vi "Attributes Setup.vi"(11 "IMAQdx Cam in":refnum<class "IMAQdx Cam.lvclass">) -> ()   [LabVIEW 2009, in "IMAQdx Cam.lvclass"]
doc: "The Grab and Attributes Setup example VI allows the user to view the current attributes and settings, update attribute settings, acquire images continuously, and display the images in an image control."
uses:
  IMAQdx Cam.lvclass
  IMAQdx Cam.lvclass/IMAQdx Cam.ctl
panel:
  in  "Filter":string
  in  "error in":errorcluster
  out "Tooltip":string
  out "Units":string
  out "Tab Control Ref":T1
  in  "Tab Control":T2(tab)
  in  "U32 Value Control":u32(slide) scale=4.0..4044.0
  in  "DBL Value Control":dbl(slide) min=17.00000029813964 max=5000000.0 step=1.0 scale=17.00000029813964..5000000.0
  in  "String Value Control":string
  in  "Enum Value Control":u32(ring) items=["Use hardware value", "10-bit", "12-bit", "14-bit", "16-bit"]
  in  "Boolean Value Control":bool=TRUE
  in  "Command Value Control":bool
  in  "Attribute Table":string(tree)
  in  "stop":bool
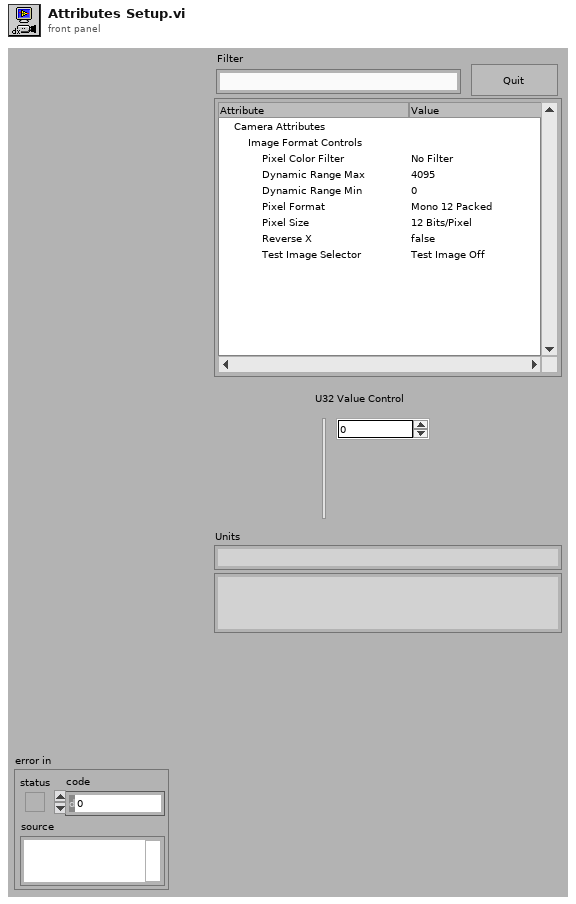
[diagram p1: front panel]
types:
  T1 = cluster{"Tab Control":refnum<vi>, "U32 Value Control":refnum<vi>, "DBL Value Control":refnum<vi>, "String Value Control":refnum<vi>, "Enum Value Control":refnum<vi>, "Boolean Value Control":refnum<vi>, "Command Value Control":refnum<vi>}
  T2 = enum32{"U32", "DBL", "String", "Enum", "Bool", "Command"}
  T3 = typedef "IMAQdx.ctl" = refnum<k21>
  T4 = typedef "eventvkey.ctl" = enum16{"ASCII", "Enter", "Return", "Shift", "Ctrl", "Alt", "Cmd", "Opt", "Caps", "NumLock", "Clear", "Break", "Up", "Down", "Left", "Right", "Insert", "Delete", "Home", "End", "PageUp", "PageDown", "Escape", "Help", "Pause", "ScrollLock", "F1", "F2", "F3", "F4", "F5", "F6", "F7", "F8", "F9", "F10", "F11", "F12", "F13", "F14", "F15", "F16", "F17", "F18", "F19", "F20", "F21", "F22", "F23", "F24", "Play", "VolumeUp", "VolumeDown", "Mute", "Two Byte Char"}
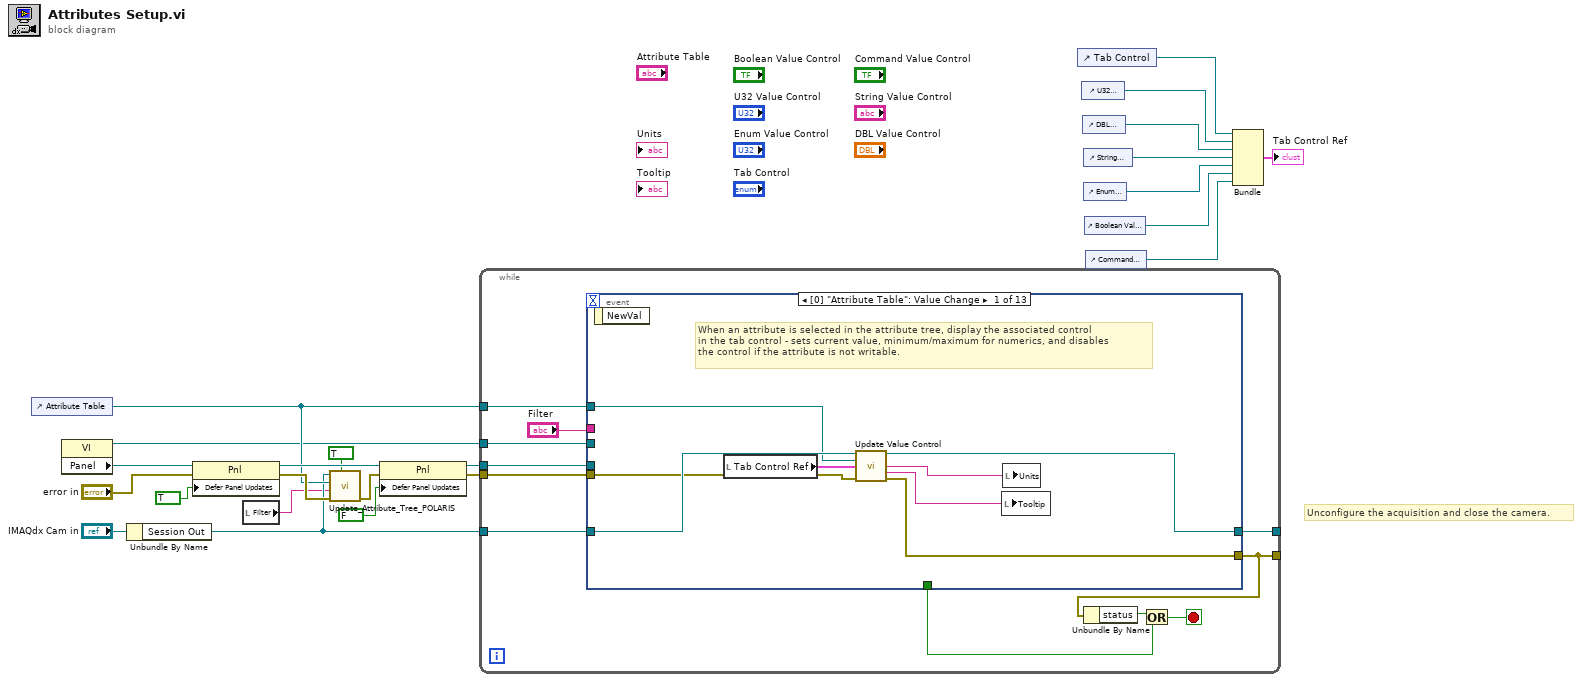
[diagram p0: block diagram]
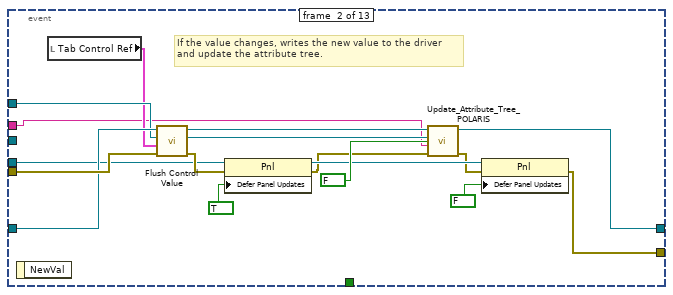
[diagram p2: hidden frame]
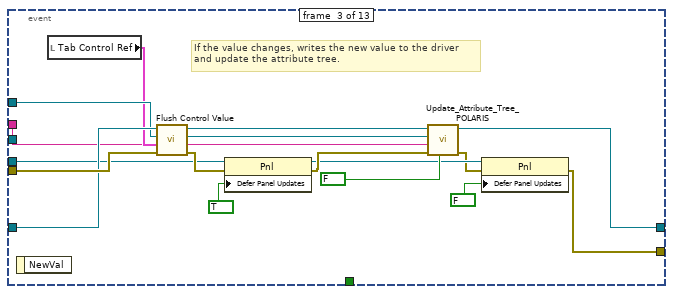
[diagram p3: hidden frame]
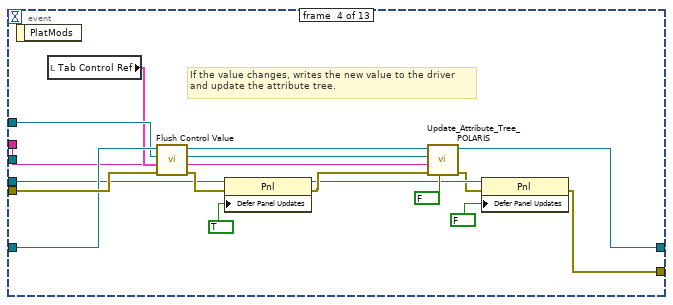
[diagram p4: hidden frame]
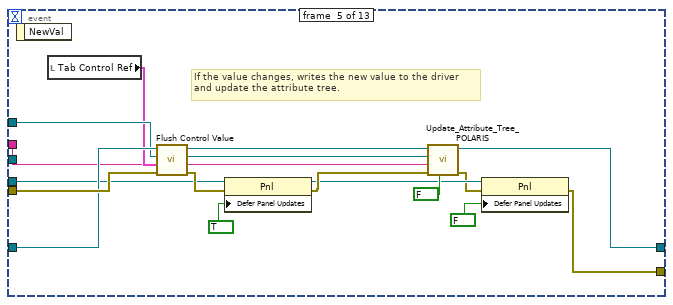
[diagram p5: hidden frame]
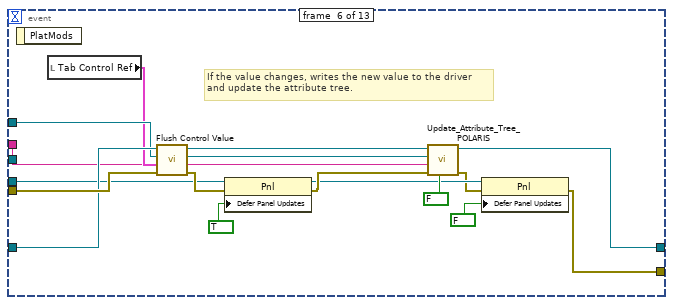
[diagram p6: hidden frame]
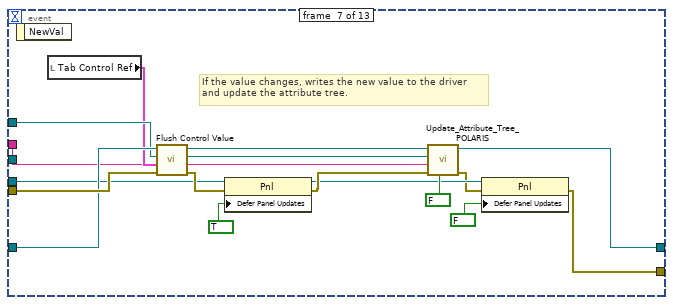
[diagram p7: hidden frame]
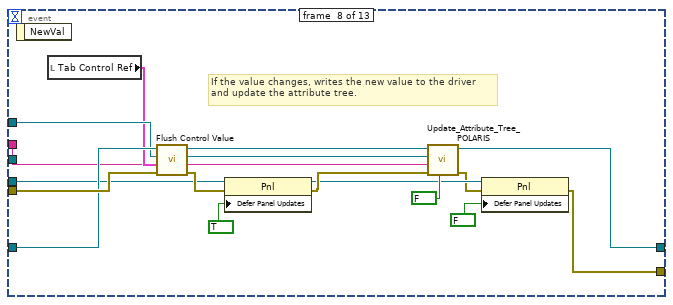
[diagram p8: hidden frame]
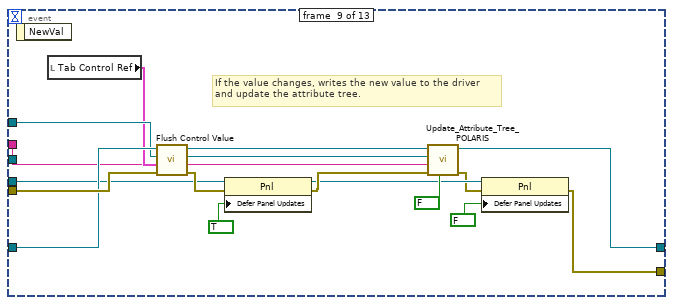
[diagram p9: hidden frame]
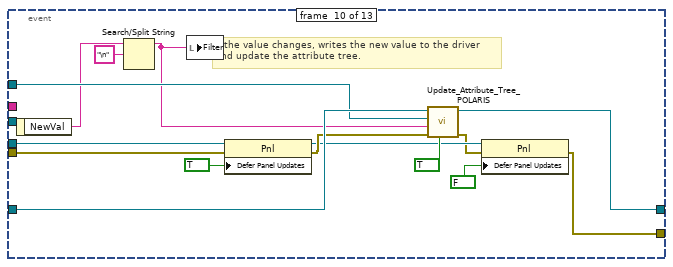
[diagram p10: hidden frame]
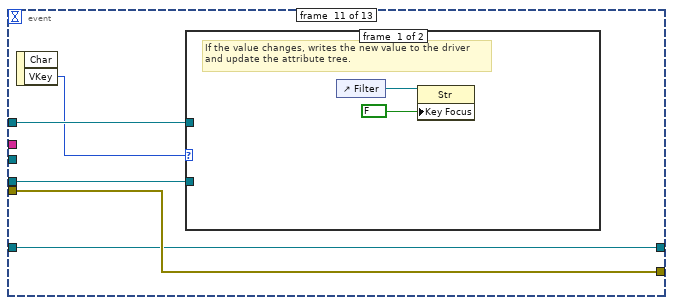
[diagram p11: hidden frame]
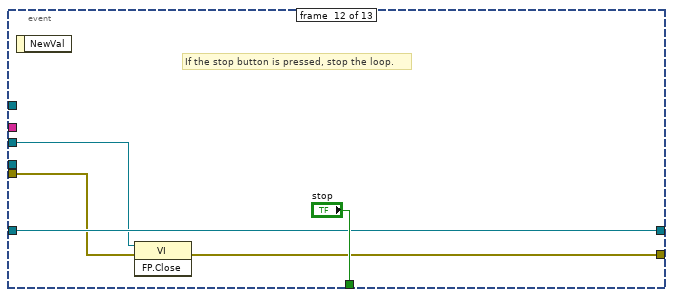
[diagram p13: hidden frame]
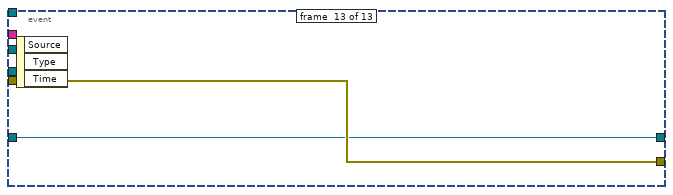
[diagram p14: hidden frame]
diagram:
  # "Unconfigure the acquisition and close the camera."
  n1 = control-ref of="Attribute Table"() -> (w11:refnum<vi>)
  n2 = property class="VI"() -> (reference out=w8:refnum<vi>, "Panel"=w9:refnum<vi>)  [unwired: 2 in, 1 out]
  n3 = Unbundle By Name("IMAQdx Cam in") -> ("Session Out"=w10:T3)
  n4 = property class="Pnl"(reference=w9, error in="error in", "Defer Panel Updates"=TRUE) -> (reference out=w12:refnum<vi>, error out=w14:errorcluster)
  n5 = local read "Filter"() -> (w2:string)
  n6 = call "Update_Attribute_Tree_POLARIS.vi"("Flush Tree?"=TRUE, "error in"=w14, "Filter"=w2, "Tree Control In"=w11, "Camera Name In"=w10) -> ("error out"=w13:errorcluster)  [unwired: 1 in, 2 out]
  n7 = property class="Pnl"(reference=w12, error in=w13, "Defer Panel Updates"=FALSE ("Flush Tree?")) -> (reference out=w7:refnum<vi>, error out=w3:errorcluster)
  n8 = while {
    tunnel: [w30] -> _
    tunnel: w3 -> [w31]
    tunnel: w10 -> [w32]
    tunnel: [w29] -> _
    tunnel: w11 -> [w28]
    tunnel: w7 -> [w27]
    tunnel: w8 -> [w25]
    stop <- w34 stop-if-true
    n9 = event shown="[0] \"Attribute Table\": Value Change" {
      selector: _ -> [_ _ _ _ _ _ _ _ _ _ _ _ _]
      dyn-events: _ -> [_ _ _ _ _ _ _ _ _ _ _ _ _]
      timeout: _ -> [_ _ _ _ _ _ _ _ _ _ _ _ _]
      tunnel: w32 -> [w42 w58 w75 w92 w109 w126 w143 w160 w177 w192 w195 w204 w206]
      tunnel: w31 -> [w40 w59 w76 w93 w110 w127 w144 w161 w178 w193 w196 w202 w207]
      tunnel: [w41 w45 w61 w78 w95 w112 w129 w146 w163 w182 w195 w204 w206] -> w30
      tunnel: [w39 w46 w62 w79 w96 w113 w130 w147 w164 w183 w196 w201 w207] -> w29
      tunnel: w28 -> [w35 w56 w73 w90 w107 w124 w141 w158 w175 w191 w198 _ _]
      tunnel: w27 -> [_ w51 w67 w84 w101 w118 w135 w152 w169 w188 w197 _ _]
      tunnel: [_ _ _ _ _ _ _ _ _ _ _ "stop" _] -> w26
      tunnel: w25 -> [_ _ _ _ _ _ _ _ _ _ _ w203 _]
      tunnel: "Filter" -> [_ w43 w60 w77 w94 w111 w128 w145 w162 _ _ _ _]
      event #0 {
        # "When an attribute is selected in the attribute tree, display the associated control\nin the tab control - sets current value, minimum/maximum for numerics, and disables\nthe control if the attribute is not writable."
        n10 = event-data() -> ()  [unwired: 2 out]
        n11 = local read "Tab Control Ref"() -> (w38:T1)
        n12 = call "Update Value Control.vi"("Session In"=w42, "Tree Control In"=w35, "Tab Control Ref In"=w38, "error in (no error)"=w40) -> ("Session Out"=w41:T3, "Units"=w37:string, "Tooltip"=w36:string, "error out"=w39:errorcluster)  [unwired: 1 in, 7 out]
        n13 = local write "Tooltip"(w36) -> ()
        n14 = local write "Units"(w37) -> ()
      }
      event #1 {
        # "If the value changes, writes the new value to the driver\nand update the attribute tree."
        n15 = event-data() -> ()  [unwired: 2 out]
        n16 = local read "Tab Control Ref"() -> (w55:T1)
        n17 = call "Flush Control Value.vi"("error in (no error)"=w59, "Tab Control Ref In"=w55, "Tree Control In"=w56, "Session In"=w58) -> ("error out"=w52:errorcluster, "Tree Control Out"=w54:refnum<vi>, "Session Out"=w57:T3)  [unwired: 1 out]
        n18 = property class="Pnl"(reference=w51, error in=w52, "Defer Panel Updates"=TRUE) -> (reference out=w49:refnum<vi>, error out=w44:errorcluster)
        n19 = call "Update_Attribute_Tree_POLARIS.vi"("Flush Tree?"=FALSE, "error in"=w44, "Filter"=w43, "Tree Control In"=w54, "Camera Name In"=w57) -> ("error out"=w48:errorcluster, "Session Out"=w45:T3)  [unwired: 1 in, 1 out]
        n20 = property class="Pnl"(reference=w49, error in=w48, "Defer Panel Updates"=FALSE) -> (error out=w46:errorcluster)  [unwired: 1 out]
      }
      event #2 {
        # "If the value changes, writes the new value to the driver\nand update the attribute tree."
        n21 = event-data() -> ()  [unwired: 2 out]
        n22 = local read "Tab Control Ref"() -> (w72:T1)
        n23 = call "Flush Control Value.vi"("error in (no error)"=w76, "Tab Control Ref In"=w72, "Tree Control In"=w73, "Session In"=w75) -> ("error out"=w68:errorcluster, "Tree Control Out"=w71:refnum<vi>, "Session Out"=w74:T3)  [unwired: 1 out]
        n24 = property class="Pnl"(reference=w67, error in=w68, "Defer Panel Updates"=TRUE) -> (reference out=w65:refnum<vi>, error out=w69:errorcluster)
        n25 = call "Update_Attribute_Tree_POLARIS.vi"("Flush Tree?"=FALSE, "error in"=w69, "Filter"=w60, "Tree Control In"=w71, "Camera Name In"=w74) -> ("error out"=w64:errorcluster, "Session Out"=w61:T3)  [unwired: 1 in, 1 out]
        n26 = property class="Pnl"(reference=w65, error in=w64, "Defer Panel Updates"=FALSE) -> (error out=w62:errorcluster)  [unwired: 1 out]
      }
      event #3 {
        # "If the value changes, writes the new value to the driver\nand update the attribute tree."
        n27 = event-data() -> ()  [unwired: 2 out]
        n28 = local read "Tab Control Ref"() -> (w89:T1)
        n29 = call "Flush Control Value.vi"("error in (no error)"=w93, "Tab Control Ref In"=w89, "Tree Control In"=w90, "Session In"=w92) -> ("error out"=w85:errorcluster, "Tree Control Out"=w88:refnum<vi>, "Session Out"=w91:T3)  [unwired: 1 out]
        n30 = property class="Pnl"(reference=w84, error in=w85, "Defer Panel Updates"=TRUE) -> (reference out=w82:refnum<vi>, error out=w86:errorcluster)
        n31 = call "Update_Attribute_Tree_POLARIS.vi"("Flush Tree?"=FALSE, "error in"=w86, "Filter"=w77, "Tree Control In"=w88, "Camera Name In"=w91) -> ("error out"=w81:errorcluster, "Session Out"=w78:T3)  [unwired: 1 in, 1 out]
        n32 = property class="Pnl"(reference=w82, error in=w81, "Defer Panel Updates"=FALSE) -> (error out=w79:errorcluster)  [unwired: 1 out]
      }
      event #4 {
        # "If the value changes, writes the new value to the driver\nand update the attribute tree."
        n33 = event-data() -> ()  [unwired: 2 out]
        n34 = local read "Tab Control Ref"() -> (w106:T1)
        n35 = call "Flush Control Value.vi"("error in (no error)"=w110, "Tab Control Ref In"=w106, "Tree Control In"=w107, "Session In"=w109) -> ("error out"=w102:errorcluster, "Tree Control Out"=w105:refnum<vi>, "Session Out"=w108:T3)  [unwired: 1 out]
        n36 = property class="Pnl"(reference=w101, error in=w102, "Defer Panel Updates"=TRUE) -> (reference out=w99:refnum<vi>, error out=w103:errorcluster)
        n37 = call "Update_Attribute_Tree_POLARIS.vi"("Flush Tree?"=FALSE, "error in"=w103, "Filter"=w94, "Tree Control In"=w105, "Camera Name In"=w108) -> ("error out"=w98:errorcluster, "Session Out"=w95:T3)  [unwired: 1 in, 1 out]
        n38 = property class="Pnl"(reference=w99, error in=w98, "Defer Panel Updates"=FALSE) -> (error out=w96:errorcluster)  [unwired: 1 out]
      }
      event #5 {
        # "If the value changes, writes the new value to the driver\nand update the attribute tree."
        n39 = event-data() -> ()  [unwired: 2 out]
        n40 = local read "Tab Control Ref"() -> (w123:T1)
        n41 = call "Flush Control Value.vi"("error in (no error)"=w127, "Tab Control Ref In"=w123, "Tree Control In"=w124, "Session In"=w126) -> ("error out"=w119:errorcluster, "Tree Control Out"=w122:refnum<vi>, "Session Out"=w125:T3)  [unwired: 1 out]
        n42 = property class="Pnl"(reference=w118, error in=w119, "Defer Panel Updates"=TRUE) -> (reference out=w116:refnum<vi>, error out=w120:errorcluster)
        n43 = call "Update_Attribute_Tree_POLARIS.vi"("Flush Tree?"=FALSE, "error in"=w120, "Filter"=w111, "Tree Control In"=w122, "Camera Name In"=w125) -> ("error out"=w115:errorcluster, "Session Out"=w112:T3)  [unwired: 1 in, 1 out]
        n44 = property class="Pnl"(reference=w116, error in=w115, "Defer Panel Updates"=FALSE) -> (error out=w113:errorcluster)  [unwired: 1 out]
      }
      event #6 {
        # "If the value changes, writes the new value to the driver\nand update the attribute tree."
        n45 = event-data() -> ()  [unwired: 2 out]
        n46 = local read "Tab Control Ref"() -> (w140:T1)
        n47 = call "Flush Control Value.vi"("error in (no error)"=w144, "Tab Control Ref In"=w140, "Tree Control In"=w141, "Session In"=w143) -> ("error out"=w136:errorcluster, "Tree Control Out"=w139:refnum<vi>, "Session Out"=w142:T3)  [unwired: 1 out]
        n48 = property class="Pnl"(reference=w135, error in=w136, "Defer Panel Updates"=TRUE) -> (reference out=w133:refnum<vi>, error out=w137:errorcluster)
        n49 = call "Update_Attribute_Tree_POLARIS.vi"("Flush Tree?"=FALSE, "error in"=w137, "Filter"=w128, "Tree Control In"=w139, "Camera Name In"=w142) -> ("error out"=w132:errorcluster, "Session Out"=w129:T3)  [unwired: 1 in, 1 out]
        n50 = property class="Pnl"(reference=w133, error in=w132, "Defer Panel Updates"=FALSE) -> (error out=w130:errorcluster)  [unwired: 1 out]
      }
      event #7 {
        # "If the value changes, writes the new value to the driver\nand update the attribute tree."
        n51 = event-data() -> ()  [unwired: 2 out]
        n52 = local read "Tab Control Ref"() -> (w157:T1)
        n53 = call "Flush Control Value.vi"("error in (no error)"=w161, "Tab Control Ref In"=w157, "Tree Control In"=w158, "Session In"=w160) -> ("error out"=w153:errorcluster, "Tree Control Out"=w156:refnum<vi>, "Session Out"=w159:T3)  [unwired: 1 out]
        n54 = property class="Pnl"(reference=w152, error in=w153, "Defer Panel Updates"=TRUE) -> (reference out=w150:refnum<vi>, error out=w154:errorcluster)
        n55 = call "Update_Attribute_Tree_POLARIS.vi"("Flush Tree?"=FALSE, "error in"=w154, "Filter"=w145, "Tree Control In"=w156, "Camera Name In"=w159) -> ("error out"=w149:errorcluster, "Session Out"=w146:T3)  [unwired: 1 in, 1 out]
        n56 = property class="Pnl"(reference=w150, error in=w149, "Defer Panel Updates"=FALSE) -> (error out=w147:errorcluster)  [unwired: 1 out]
      }
      event #8 {
        # "If the value changes, writes the new value to the driver\nand update the attribute tree."
        n57 = event-data() -> ()  [unwired: 2 out]
        n58 = local read "Tab Control Ref"() -> (w174:T1)
        n59 = call "Flush Control Value.vi"("error in (no error)"=w178, "Tab Control Ref In"=w174, "Tree Control In"=w175, "Session In"=w177) -> ("error out"=w170:errorcluster, "Tree Control Out"=w173:refnum<vi>, "Session Out"=w176:T3)  [unwired: 1 out]
        n60 = property class="Pnl"(reference=w169, error in=w170, "Defer Panel Updates"=TRUE) -> (reference out=w167:refnum<vi>, error out=w171:errorcluster)
        n61 = call "Update_Attribute_Tree_POLARIS.vi"("Flush Tree?"=FALSE, "error in"=w171, "Filter"=w162, "Tree Control In"=w173, "Camera Name In"=w176) -> ("error out"=w166:errorcluster, "Session Out"=w163:T3)  [unwired: 1 in, 1 out]
        n62 = property class="Pnl"(reference=w167, error in=w166, "Defer Panel Updates"=FALSE) -> (error out=w164:errorcluster)  [unwired: 1 out]
      }
      event #9 {
        # "If the value changes, writes the new value to the driver\nand update the attribute tree."
        n63 = event-data() -> ("NewVal"=w181:string)  [unwired: 1 out]
        n64 = Search/Split String(string=w181, search string/char (-)="\n") -> (substring before match=w179:string)  [unwired: 1 in, 2 out]
        n65 = local write "Filter"(w179) -> ()
        n66 = property class="Pnl"(reference=w188, error in=w193, "Defer Panel Updates"=TRUE) -> (reference out=w186:refnum<vi>, error out=w189:errorcluster)
        n67 = call "Update_Attribute_Tree_POLARIS.vi"("Flush Tree?"=TRUE, "error in"=w189, "Filter"=w179, "Tree Control In"=w191, "Camera Name In"=w192) -> ("error out"=w185:errorcluster, "Session Out"=w182:T3)  [unwired: 1 in, 1 out]
        n68 = property class="Pnl"(reference=w186, error in=w185, "Defer Panel Updates"=FALSE) -> (error out=w183:errorcluster)  [unwired: 1 out]
      }
      event #10 {
        n69 = event-data() -> ("VKey"=w194:T4)  [unwired: 2 out]
        n70 = case shown="\"Return\"" w194 {
          tunnel: w198 -> [_ _]
          tunnel: w197 -> [_ _]
          frame #0 {
            # "If the value changes, writes the new value to the driver\nand update the attribute tree."
            n71 = control-ref of="Filter"() -> (w199:refnum<vi>)
            n72 = property class="Str"(reference=w199, "Key Focus"=FALSE) -> ()  [unwired: 1 in, 2 out]
          }
          frame #1 {
          }
        }
      }
      event #11 {
        # "If the stop button is pressed, stop the loop."
        n73 = event-data() -> ()  [unwired: 2 out]
        n74 = invoke class="VI" method="FP.Close"(reference=w203, error in=w202) -> (error out=w201:errorcluster)  [unwired: 1 in, 2 out]
      }
      event #12 {
        n75 = event-data() -> ()  [unwired: 4 out]
      }
    }
    n76 = Unbundle By Name(w29) -> ("status"=w33:bool)
    n77 = Or(x=w33, y=w26) -> (x .or. y?=w34:bool)
  }
  n78 = control-ref of="Tab Control"() -> (w23:refnum<vi>)
  n79 = control-ref of="U32 Value Control"() -> (w21:refnum<vi>)
  n80 = control-ref of="DBL Value Control"() -> (w20:refnum<vi>)
  n81 = control-ref of="String Value Control"() -> (w22:refnum<vi>)
  n82 = control-ref of="Enum Value Control"() -> (w19:refnum<vi>)
  n83 = control-ref of="Boolean Value Control"() -> (w18:refnum<vi>)
  n84 = control-ref of="Command Value Control"() -> (w17:refnum<vi>)
  n85 = Bundle("Tab Control"=w23, "U32 Value Control"=w21, "DBL Value Control"=w20, "String Value Control"=w22, "Enum Value Control"=w19, "Boolean Value Control"=w18, "Command Value Control"=w17) -> (→"Tab Control Ref":T1)  [unwired: 1 out]
